vi "Vision - Get Panel Bounds.vi"(8 "error in (no error)":errorcluster, 11 "VI in":refnum<vi>) -> (0 "error out":errorcluster, 2 "Panel Size":T1, 3 "Panel Bounds":T2)   [LabVIEW 2024]
uses:
  <vilib>/Utility/miscctls.llb/LVRectTypeDef.ctl
  <vilib>/Utility/miscctls.llb/LVBoundsTypeDef.ctl
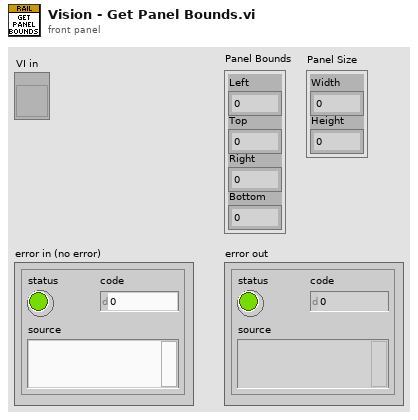
[diagram p1: front panel]
types:
  T1 = typedef "LVBoundsTypeDef.ctl" = cluster{"Width":u32, "Height":u32}
  T2 = typedef "LVRectTypeDef.ctl" = cluster{"Left":i16, "Top":i16, "Right":i16, "Bottom":i16}
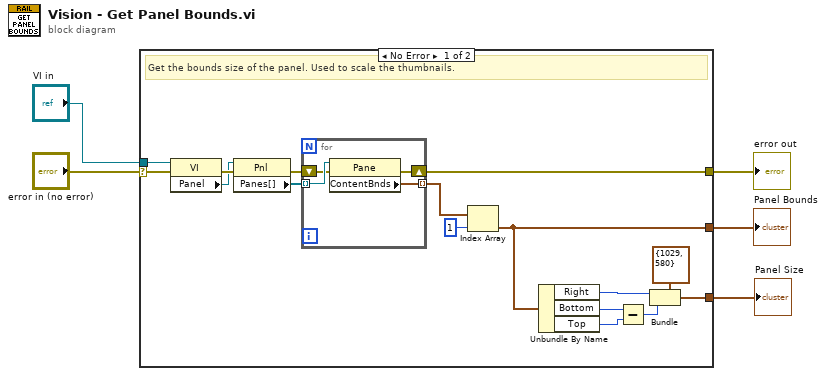
[diagram p0: block diagram]
diagram:
  n1 = case shown="No Error" "error in (no error)" {
    selector: "error in (no error)" -> [w13 w26]
    tunnel: [w21 w26] -> w5
    tunnel: [w7 _] -> w4
    tunnel: "VI in" -> [w14 _]
    tunnel: [w6 _] -> w1
    frame No Error {
      # "Get the bounds size of the panel. Used to scale the thumbnails."
      n2 = property class="VI"(reference=w14, error in=w13) -> (error out=w19:errorcluster, "Panel"=w15:refnum<vi>)  [unwired: 1 out]
      n3 = property class="Pnl"(reference=w15, error in=w19) -> (error out=w20:errorcluster, "Panes[]"=w16:refnum<vi>[])  [unwired: 1 out]
      n4 = for {
        tunnel: w16 -> [w25] mode=indexing
        tunnel: [w24] -> w17 mode=indexing
        shift-right: [w22] -> w21
        shift-left: w20 -> [w23]
        n5 = property on="Property Node" class="Pane"(reference=w25, error in=w23) -> (error out=w22:errorcluster, "ContentBnds"=w24:T2)  [unwired: 1 out]
      }
      n6 = Index Array(array=w17, index=1) -> (element=w7:T2)
      n7 = Unbundle By Name(w7) -> ("Right"=w11:i16, "Bottom"=w10:i16, "Top"=w8:i16)
      n8 = Subtract(x=w10, y=w8) -> (x-y=w9:i16)
      n9 = Bundle(cluster=T1 {"Width"=1029, "Height"=580} ("Bounds"), "Width"=w11, "Height"=w9) -> (w6:T1)
    }
    frame Error {
    }
  }
  "error out" <- w5
  "Panel Bounds" <- w4
  "Panel Size" <- w1
